vi "GetSystemTimeZones.vi"(11 "Error in":errorcluster caption="Error in (no error)") -> (4 "System Timezone Names":string[](array[string]), 6 "System Timezone Descriptors":string[](array[string]), 8 "UTC Offsets":dbl[](array[numeric]), 15 "Error out":errorcluster)   [LabVIEW 2017, in "GPTiming.lvlib"]
doc: "Queries the (Windows only) system for available timezones.\n\n<B>System Timezone Descriptors</B> can be used in a listbox to allow a user to select a time zone, while the corresponding entries in either <B>System Timezone Names</B> or <B>UTC Offsets</B> must be used when setting a new timezone.\n\nThis VI runs only if there is no error on <B>Error in</B>.\n\nSteen Schmidt\nGPower\n4/2 2017"
uses:
  GPTiming.lvlib
  Error/GPError.lvlib
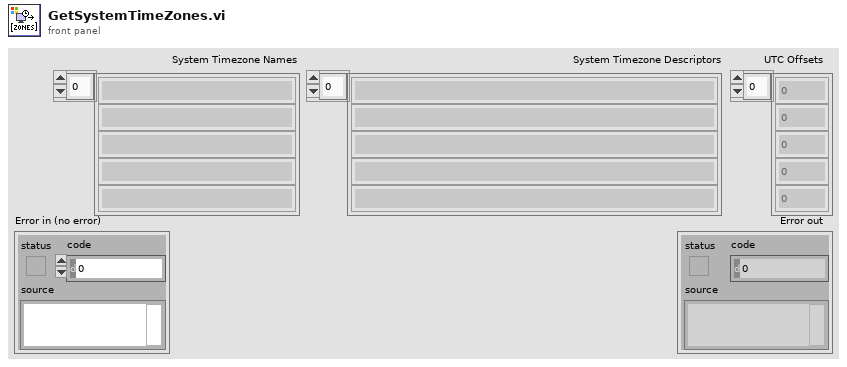
[diagram p1: front panel]
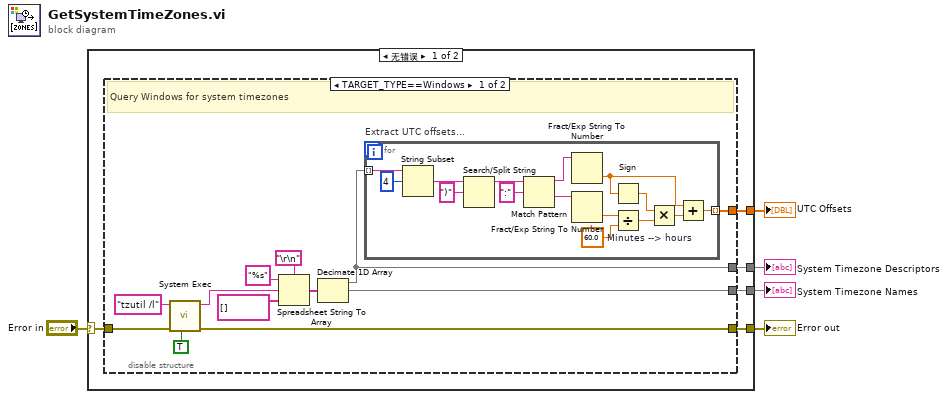
[diagram p0: block diagram]
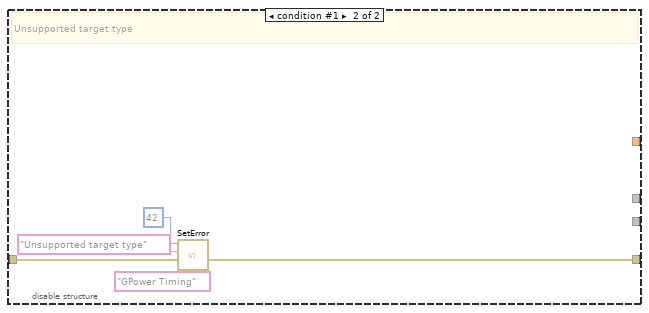
[diagram p2: hidden frame]
diagram:
  n1 = case shown="无错误" "Error in" {
    selector: "Error in" -> [w10 w43]
    tunnel: [w9 w43] -> w5
    tunnel: [w8 _] -> w4
    tunnel: [w7 _] -> w3
    tunnel: [w6 _] -> w2
    frame No Error {
      n2 = disable-structure shown="TARGET_TYPE==Windows" {
        disable-tunnel: w10 -> [w15 w40]
        disable-tunnel: [w14 w38] -> w9
        disable-tunnel: [w13 _] -> w8
        disable-tunnel: [w12 _] -> w7
        disable-tunnel: [w11 _] -> w6
        frame condition #0 (active) {
          # "Query Windows for system timezones"
          n3 = call <vilib>:"System Exec.vi"("run minimized? (F)"=TRUE, "error in (no error)"=w15, "command line"="tzutil /l") -> ("error out"=w14:errorcluster, "standard output"=w18:string)  [unwired: 5 in, 2 out]
          n4 = Spreadsheet String To Array(delimiter (Tab)="\r\n", format string="%s", spreadsheet string=w18, array type (2D Dbl)=string[] []) -> (array=w22:string[])
          n5 = Decimate 1D Array(w22) -> (w12:string[], w13:string[])  [unwired: 1 out]
          n6 = for "Extract UTC offsets..." {
            tunnel: w12 -> [w36] mode=indexing
            tunnel: [w27] -> w11 mode=indexing
            w28 = 60.0  # Minutes --> hours
            n7 = String Subset(string=w36, offset (0)=4) -> (substring=w35:string)  [unwired: 1 in]
            n8 = Search/Split String(string=w35, search string/char (-)=")") -> (substring before match=w33:string)  [unwired: 1 in, 2 out]
            n9 = Match Pattern(string=w33, regular expression=":") -> (before substring=w31:string, after substring=w30:string)  [unwired: 1 in, 2 out]
            n10 = Fract/Exp String To Number(string=w31) -> (number=w26:dbl)  [unwired: 3 in, 1 out]
            n11 = Fract/Exp String To Number(string=w30) -> (number=w29:dbl)  [unwired: 3 in, 1 out]
            n12 = Sign(1:w26) -> (0:w23:dbl)
            n13 = Divide(x=w29, y=w28) -> (x/y=w25:dbl)
            n14 = Multiply(x=w23, y=w25) -> (x*y=w24:dbl)
            n15 = Add(x=w26, y=w24) -> (x+y=w27:dbl)
          }
        }
        frame condition #1 {
          # "Unsupported target type"
          n16 = call "SetError.vi"("Error label"="GPower Timing", "Error in"=w40, "Error description"="Unsupported target type", "Error code"=42) -> ("Error out"=w38:errorcluster)  [unwired: 7 in]
        }
      }
    }
    frame Error {
    }
  }
  "Error out" <- w5
  "System Timezone Descriptors" <- w3
  "System Timezone Names" <- w4
  "UTC Offsets" <- w2
